vi "Status_Demo.vi"() -> ()   [LabVIEW 2015]
panel:
  out "Longitude":string
  out "Latitude":string
  out "Time (24h)":string
  out "Manual Set Temp (C)":string
  in  "Port":string
  in  "IP":string
  out "Date":string
  out "Temperature (C)":string
  out "Status All":string
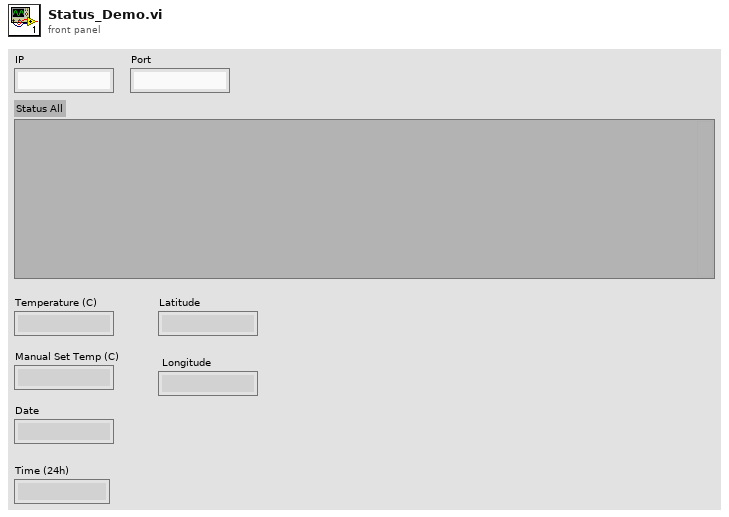
[diagram p1: front panel]
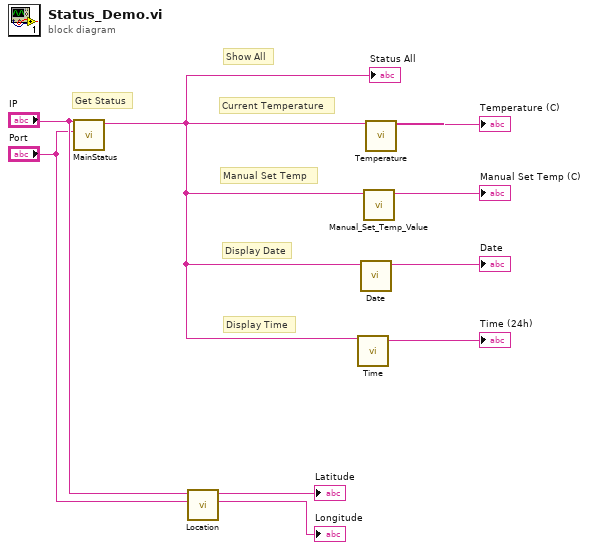
[diagram p0: block diagram]
diagram:
  # "Get Status"
  # "Current Temperature"
  # "Display Time"
  # "Display Date"
  # "Manual Set Temp"
  # "Show All"
  n1 = call "MainStatus.vi"("Port"="Port", "IP"="IP") -> ("Output All"=w9:string)  [unwired: 9 in]
  "Status All" <- w9
  n2 = call "Location.vi"("Port in"="Port", "IP in"="IP") -> ("Longitude"=→"Longitude":string, "Latitude"=→"Latitude":string)  [unwired: 8 in]
  n3 = call "Time.vi"("Output All"=w9) -> ("Time (24h)"=→"Time (24h)":string)  [unwired: 10 in]
  n4 = call "Date.vi"("Output All"=w9) -> ("Date"=→"Date":string)  [unwired: 10 in]
  n5 = call "Manual_Set_Temp_Value.vi"("Output All"=w9) -> ("Manual Set Temp (C)"=→"Manual Set Temp (C)":string)  [unwired: 10 in]
  n6 = call "Temperature.vi"("Output All"=w9) -> ("Temperature (C)"=→"Temperature (C)":string)  [unwired: 10 in]
